vi "Dispose.vi"(8 "error in":errorcluster, 11 "NYPizzaStore":refnum<class "NYPizzaStore.lvclass">) -> (0 "error out":errorcluster)   [LabVIEW 2020, in "FactoryMethod.lvlib" / "PizzaFactoryMethod.lvlib" / "NYPizzaStore.lvclass"]
uses:
  NYPizzaStore.lvclass
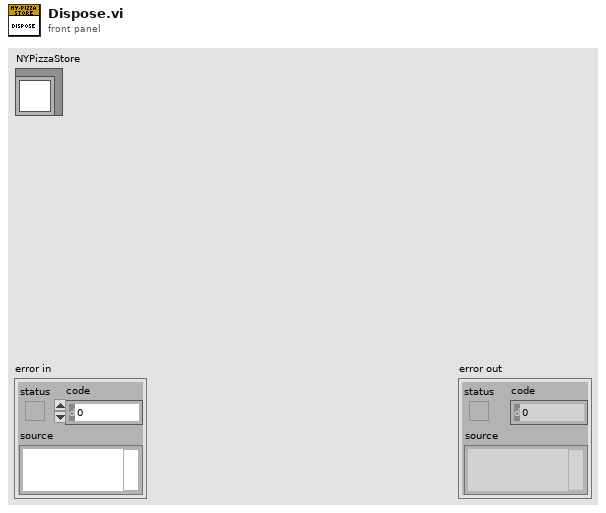
[diagram p1: front panel]
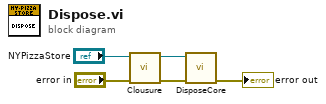
[diagram p0: block diagram]
diagram:
  n1 = call-dynamic "Clousure.vi"("error in (no error)"="error in", "NYPizzaStore"="NYPizzaStore") -> ("error out"=w3:errorcluster, "NYPizzaStore"=w4:refnum<class "NYPizzaStore.lvclass">)  [unwired: 8 in]
  n2 = call-dynamic "DisposeCore.vi"("error in (no error)"=w3, "NYPizzaStore"=w4) -> ("error out"=→"error out":errorcluster)  [unwired: 8 in, 1 out]
